vi "Logger Set Server Run Mode.vi"(0 "Server Status":enum16{"Running", "Closed"}(ring), 11 "error in (no error)":errorcluster) -> (15 "error out":errorcluster)   [LabVIEW 2018]
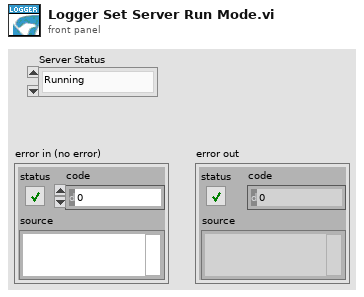
[diagram p1: front panel]
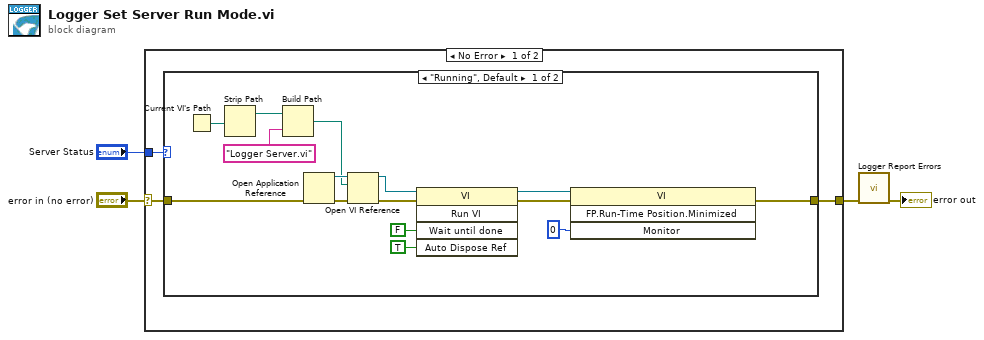
[diagram p0: block diagram]
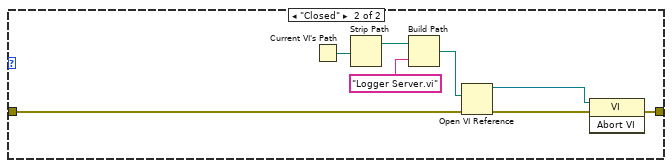
[diagram p2: hidden frame]
diagram:
  n1 = case shown="No Error" "error in (no error)" {
    selector: "error in (no error)" -> [w7 w31]
    tunnel: [w6 w31] -> w2
    tunnel: "Server Status" -> [w5 _]
    frame No Error {
      n2 = case shown="\"Running\", Default" w5 {
        tunnel: w7 -> [w22 w28]
        tunnel: [w13 w27] -> w6
        frame "Running", Default {
          n3 = Current VI's Path() -> (path=w11:path)
          n4 = Strip Path(path=w11) -> (stripped path=w10:path)  [unwired: 1 out]
          n5 = Build Path(base path=w10, name or relative path="Logger Server.vi") -> (appended path=w8:path)
          n6 = Open Application Reference(8:w22) -> (0:w20:errorcluster, 3:w21:refnum<vi>)  [unwired: 3 in]
          n7 = Open VI Reference(application reference (local)=w21, vi path=w8, error in (no error)=w20) -> (vi reference=w18:refnum<vi>, error out=w19:errorcluster)  [unwired: 3 in]
          n8 = invoke class="VI" method="Run VI"(reference=w18, error in=w19, "Wait until done"=FALSE ("Wait Until Done"), "Auto Dispose Ref"=TRUE ("Auto Dispose Reference")) -> (reference out=w17:refnum<vi>, error out=w16:errorcluster)  [unwired: 1 in, 3 out]
          n9 = invoke class="VI" method="FP.Run-Time Position.Minimized"(reference=w17, error in=w16, "Monitor"=i16 0) -> (error out=w13:errorcluster)  [unwired: 1 in, 3 out]
        }
        frame "Closed" {
          n10 = Current VI's Path() -> (path=w26:path)
          n11 = Strip Path(path=w26) -> (stripped path=w25:path)  [unwired: 1 out]
          n12 = Build Path(base path=w25, name or relative path="Logger Server.vi") -> (appended path=w23:path)
          n13 = Open VI Reference(vi path=w23, error in (no error)=w28) -> (vi reference=w29:refnum<vi>, error out=w30:errorcluster)  [unwired: 4 in]
          n14 = invoke class="VI" method="Abort VI"(reference=w29, error in=w30) -> (error out=w27:errorcluster)  [unwired: 1 in, 2 out]
        }
      }
    }
    frame Error {
    }
  }
  n15 = call "Logger Report Errors.vi"("error in (no error)"=w2) -> ("error out"=→"error out":errorcluster)  [unwired: 14 in]
